vi "Get Addresses for Measurements.vi"(8 "error in (no error)":errorcluster, 10 "config file refnum in":T1, 11 "IED in":refnum<class "IED.lvclass">) -> (0 "error out":errorcluster, 2 "config file refnum out":T1, 3 "IED out":refnum<class "IED.lvclass">)   [LabVIEW 2015, in "IED Actor.lvlib" / "IED.lvclass"]
uses:
  IED.lvclass
  <vilib>/Utility/config.llb/Config Data RefNum.ctl
  IED.lvclass/IED.ctl
  <vilib>/NI/Tools/Keyed Array/Map String.vi
  <vilib>/NI/Tools/String/Get Case Matching.vi
  <vilib>/Utility/config.llb/Read Key (U32).vi
  <vilib>/NI/Tools/Keyed Array/Tools_KeyedArray.lvlib
  <vilib>/Utility/config.llb/NI_LVConfig.lvlib
  Utilities/Message Strings.llb/Message String Utilities.lvlib
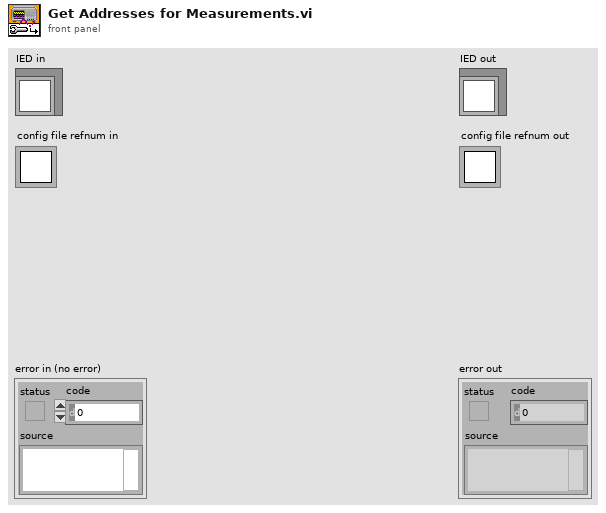
[diagram p1: front panel]
types:
  T1 = typedef "NI_LVConfig.lvlib/Config Data RefNum.ctl" = refnum<k1>
  T2 = typedef "Tools_KeyedArray.lvlib/KeyedArray.ctl" = cluster{"keys":string[], "values":string[]}
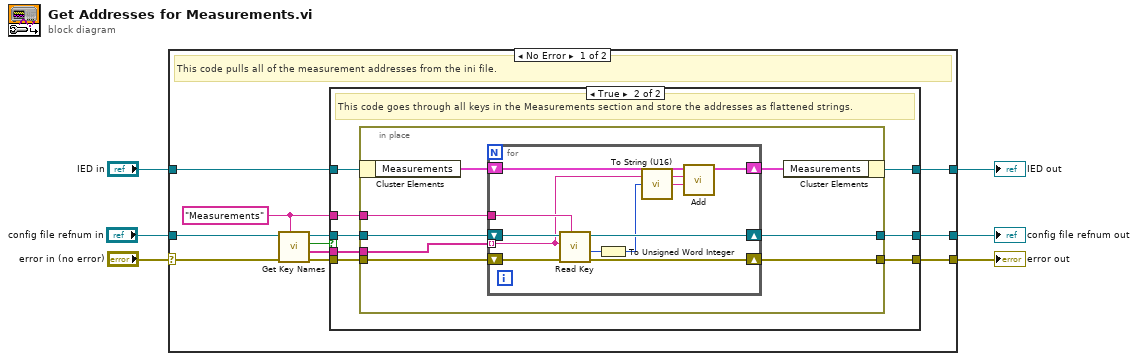
[diagram p0: block diagram]
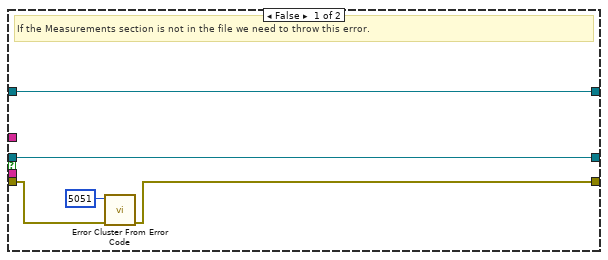
[diagram p2: hidden frame]
diagram:
  n1 = case shown="No Error" "error in (no error)" {
    selector: "error in (no error)" -> [w14 w52]
    tunnel: [w17 w52] -> w5
    tunnel: [w16 w51] -> w3
    tunnel: "IED in" -> [w7 w51]
    tunnel: "config file refnum in" -> [w15 w50]
    tunnel: [w9 w50] -> w1
    frame No Error {
      w8 = "Measurements" ("section")
      # "This code pulls all of the measurement addresses from the ini file."
      n2 = call <vilib>:"Get Key Names.vi"("section"=w8, "error in (no error)"=w14, "refnum"=w15) -> ("error out"=w10:errorcluster, "key names"=w11:string[], "section exists?"=w13:bool, "refnum out"=w12:T1)  [unwired: 5 in]
      n3 = case shown="True" w13 {
        tunnel: w7 -> [w19 w30]
        tunnel: [w20 w29] -> w17
        tunnel: [w19 w28] -> w16
        tunnel: w12 -> [w18 w25]
        tunnel: w11 -> [_ w26]
        tunnel: w10 -> [w22 w27]
        tunnel: [w18 w23] -> w9
        tunnel: w8 -> [_ w24]
        frame False {
          # "If the Measurements section is not in the file we need to throw this error."
          n4 = call <vilib>:"Error Cluster From Error Code.vi"("error in (no error)"=w22, "error code (0)"=5051) -> ("error out"=w20:errorcluster)  [unwired: 7 in]
        }
        frame True {
          # "This code goes through all keys in the Measurements section and store the addresses as flattened strings."
          n5 = in-place {
            in-place-border: [w38] -> w29
            in-place-border: w27 -> [w35]
            in-place-border: w26 -> [w34]
            in-place-border: w25 -> [w33]
            in-place-border: w24 -> [w32]
            in-place-border: [w31] -> w23
            n6 = in-place-cluster #1(w30) -> ("Measurements"=w37:T2)
            n7 = for {
              shift-right: [w43] -> w38
              shift-left: w35 -> [w46]
              shift-right: [w48] -> w36
              shift-left: w37 -> [w49]
              tunnel: w34 -> [w39] mode=indexing
              tunnel: w32 -> [w45]
              shift-right: [w44] -> w31
              shift-left: w33 -> [w47]
              n8 = call-poly <vilib>:"Read Key.vi"("section"=w45, "error in (no error)"=w46, "key"=w39, "refnum"=w47) -> ("error out"=w43:errorcluster, "value"=w42:u32, "refnum out"=w44:T1)  [unwired: 4 in, 1 out]
              n9 = To Unsigned Word Integer(number=w42) -> (unsigned 16bit integer=w40:u16)
              n10 = call "To String (U16).vi"("UINT16 in"=w40) -> ("String out"=w41:string)
              n11 = call <vilib>:"Add.vi"("value"=w41, "key"=w39, "array in"=w49) -> ("array out"=w48:T2)  [unwired: 2 in, 2 out]
            }
            n12 = in-place-cluster #1("Measurements"=w36) -> (w28:refnum<class "IED.lvclass">)
          }
        }
      }
    }
    frame Error {
    }
  }
  "error out" <- w5
  "IED out" <- w3
  "config file refnum out" <- w1
